vi "ep_EN50160 Basic Statistical Evaluation.vi"   [LabVIEW 2011, in "NI_EP_Power Quality.lvlib"]
uses:
  <vilib>/addons/Electrical Power/PQ/NI_EP_Power Quality.lvlib
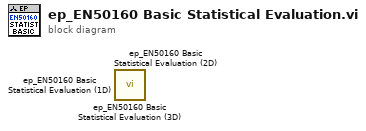
[diagram p0: block diagram]
diagram:
  n1 = call <vilib>:"ep_EN50160 Basic Statistical Evaluation (3D).vi"() -> ()  [unwired: 13 in, 3 out]
  n2 = call <vilib>:"ep_EN50160 Basic Statistical Evaluation (2D).vi"() -> ()  [unwired: 13 in, 3 out]
  n3 = call <vilib>:"ep_EN50160 Basic Statistical Evaluation (1D).vi"() -> ()  [unwired: 13 in, 3 out]
